vi "loop.vi"() -> ()   [LabVIEW 2018]
panel:
  out "number (0 to 1)":dbl(graph)
  in  "stop":bool
  out "Numeric":i32
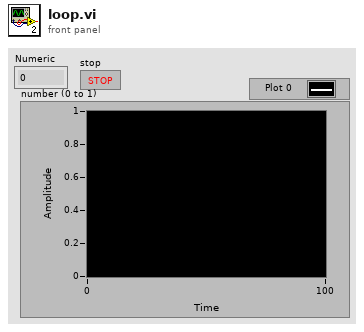
[diagram p1: front panel]
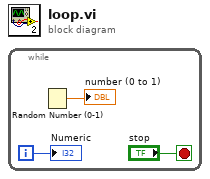
[diagram p0: block diagram]
diagram:
  n1 = while {
    i -> [w3]
    stop <- "stop" stop-if-true
    n2 = Random Number (0-1)() -> (number: 0 to 1=→"number (0 to 1)":dbl)
    "Numeric" <- w3
  }
